vi "Aquiring a Signal.vi"() -> ()   [LabVIEW 2020]
doc: "Use this template to simulate the generation and display of data.\nNote: LabVIEW enables automatic error handling by default for VIs you create from this template."
uses:
  Instance           1 27Saved   GenerateDisplay.vit .vi
  <vilib>/express/express shared/transition.llb/Dynamic To Waveform Array.vi
  <vilib>/express/express arith-compare/Formula/Block/exnFormulaBlock how many pts in the wave.vi
  <vilib>/express/express shared/ex_Modify Signal Name.vi
  <vilib>/express/express shared/transition.llb/Waveform Array To Dynamic.vi
  <vilib>/express/express arith-compare/Formula/XNode/ExpressFormulaBlockNode.xnode
panel:
  out "Table":string[][](table)
  in  "Dial":dbl(knob) scale=0.0..10.0
  in  "Knob":dbl(knob) scale=0.0..10.0
  out "Waveform Chart":dynamicdata(graph)
  out "Waveform Graph":dynamicdata(graph)
  in  "stop":bool
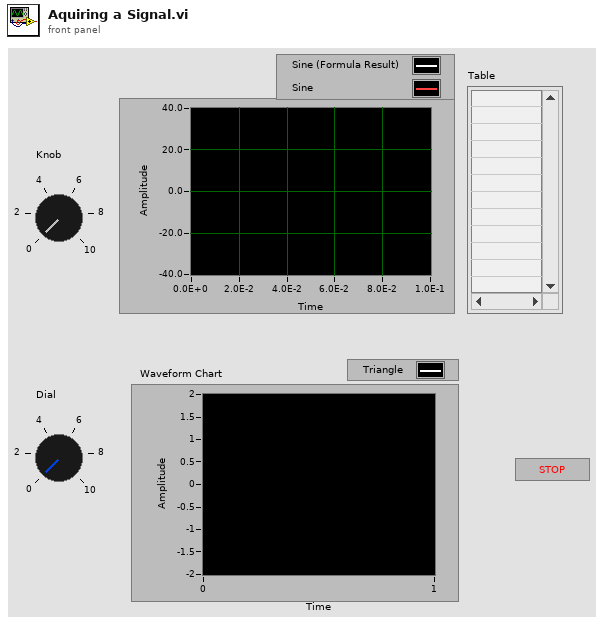
[diagram p1: front panel]
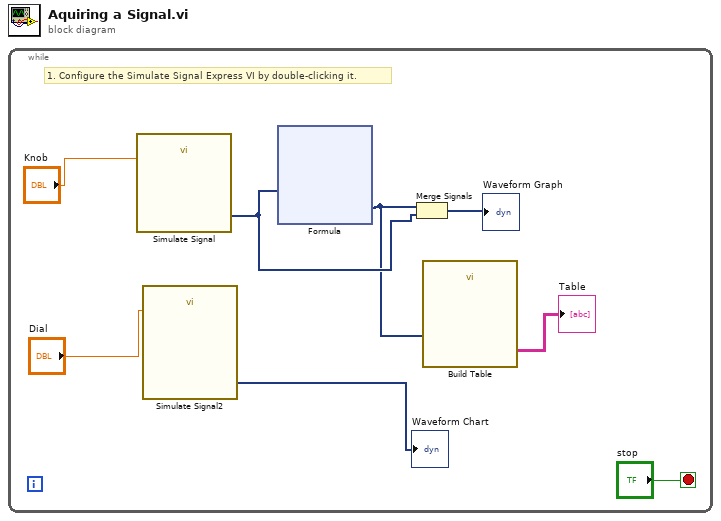
[diagram p0: block diagram]
diagram:
  n1 = while {
    stop <- "stop" stop-if-true
    # "1. Configure the Simulate Signal Express VI by double-clicking it."
    n2 = call "Simulate Signal"("Amplitude"="Knob") -> ("Sine"=w2:dynamicdata)  [unwired: 13 in, 1 out]
    n3 = call "Simulate Signal2"("Amplitude"="Dial") -> ("Triangle"=→"Waveform Chart":dynamicdata)  [unwired: 13 in, 1 out]
    n4 = xnode "Formula"("X1"=w2) -> ("Result"=w1:dynamicdata)  [unwired: 1 in, 1 out]
    n5 = Merge Signals(w1, w2) -> (→"Waveform Graph":dynamicdata)
    n6 = call "Build Table"("Signals"=w1) -> ("Table"=→"Table":string[][])  [unwired: 4 in, 6 out]
  }
